vi "Add BPP Test Results Data new.vi"(8 "error in (no error)":errorcluster, 10 "Collimation Data":T1, 11 "Test in":refnum<k24>) -> (0 "error out":errorcluster, 3 "Test out":refnum<k24>)   [LabVIEW 2018]
uses:
  C:/Program Files (x86)/National Instruments/LabVIEW 2018/user.lib/nEQdb_DLL/NEQdbAPI.dll
  Program Files (x86)/National Instruments/LabVIEW 2018/user.lib/nEQdb_DLL/NEQdbAPI.dll
  State data/Records.ctl
  0415c7d9-6818-4349-a3d2-afeb8a82f6ab.vi
  0415c7d9-6818-4349-a3d2-afeb8a82f6ab.vi/6e08599f-9911-4127-abcd-496574c18721.vi
panel:
  in  "BPP items to save":T2(ring)
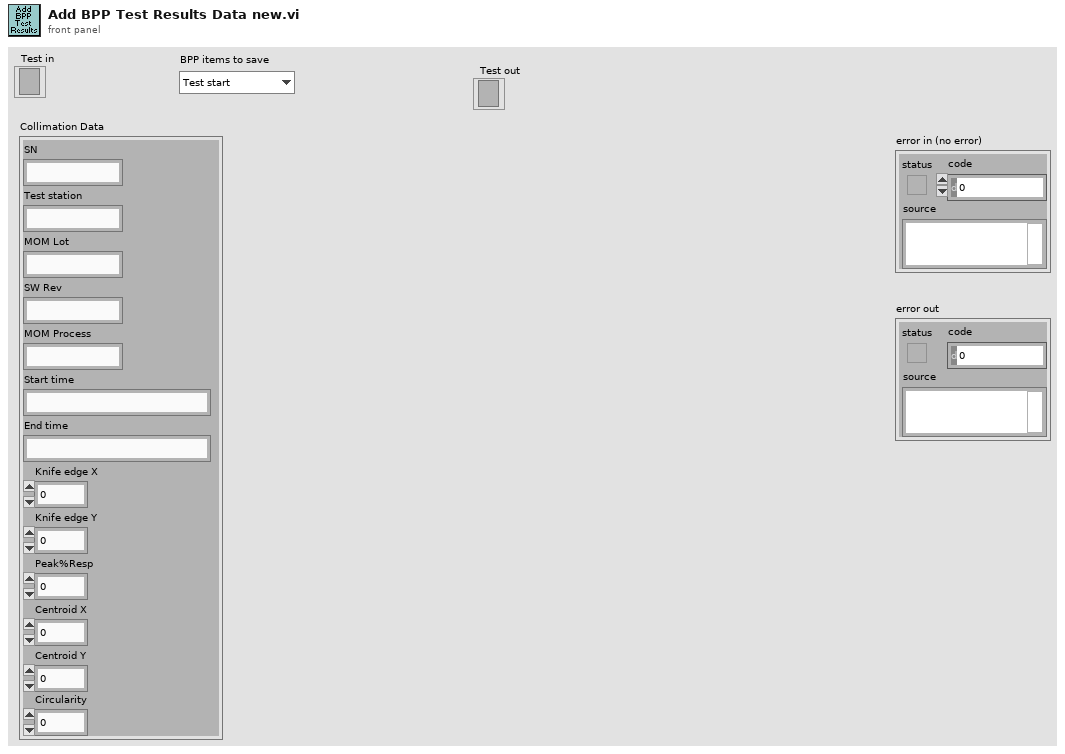
[diagram p1: front panel]
types:
  T1 = typedef "Records.ctl" = cluster{"SN":string, "Test station":string, "MOM Lot":string, "SW Rev":string, "MOM Process":string, "Start time":string, "End time":string, "Knife edge X":dbl, "Peak%Resp":dbl, "Centroid X":dbl, "Knife edge Y":dbl, "Centroid Y":dbl, "Circularity":dbl}
  T2 = enum16{"Test start", "Test finish", "FF Peak Response", "Ellipticity", "MeasuredCentroidX", "MeasuredCentroidY", "BeamViewKnifeEdge84PctX", "BeamViewKnifeEdge84PctY"}
  T3 = enum16{"Test start", "Test finish", "FF Peak Response", "Ellipticity", "MeasuredCentroidX", "MeasuredCentroidY", "BeamViewKnifeEdge84PctX", "BeamViewKnifeEdge84PctY"}[]
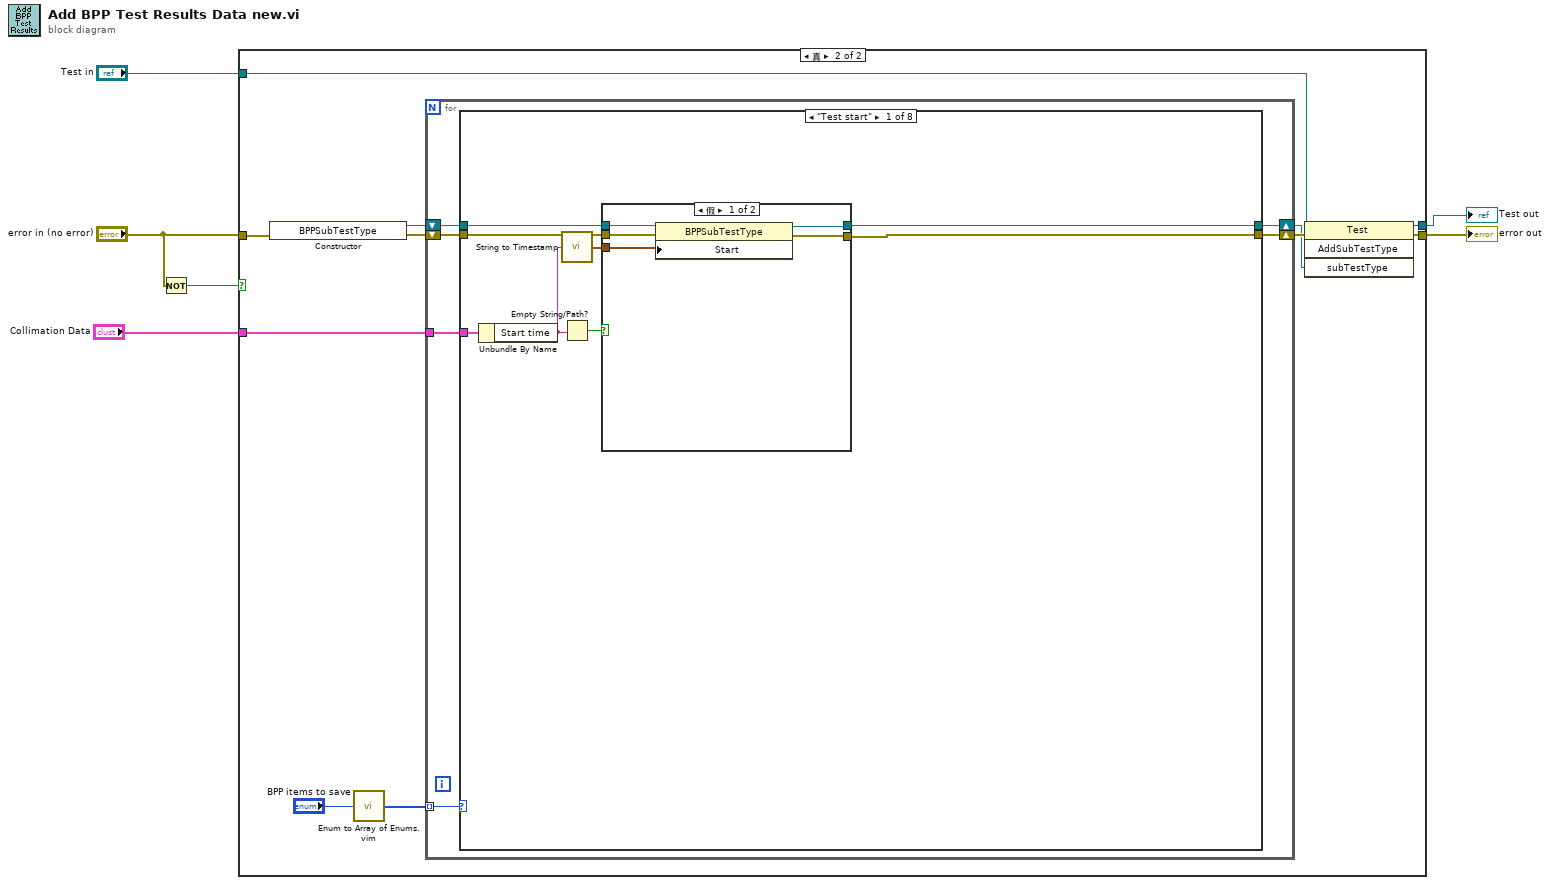
[diagram p0: block diagram]
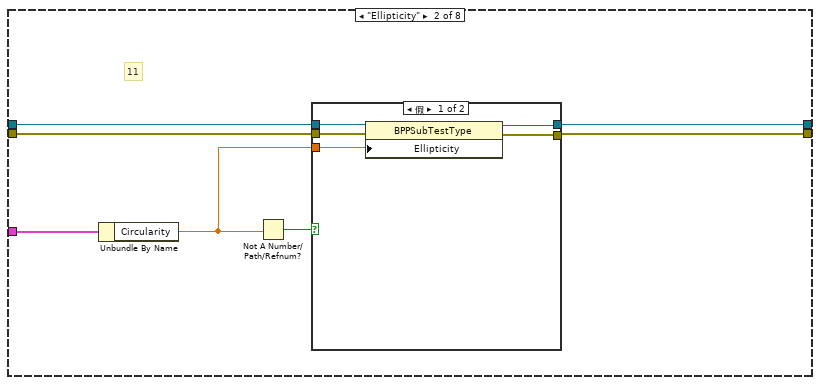
[diagram p4: hidden frame]
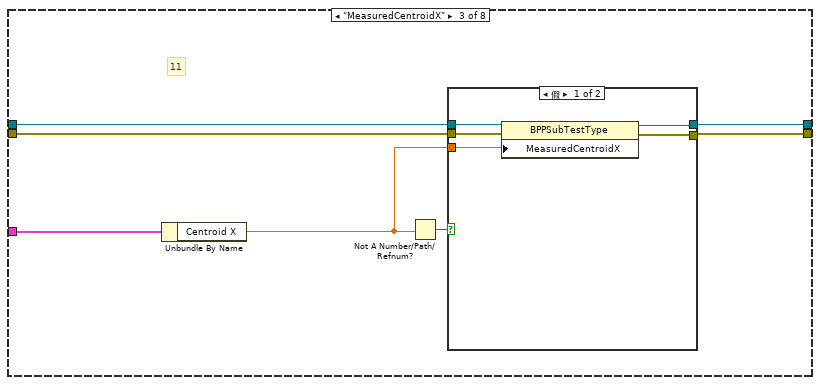
[diagram p6: hidden frame]
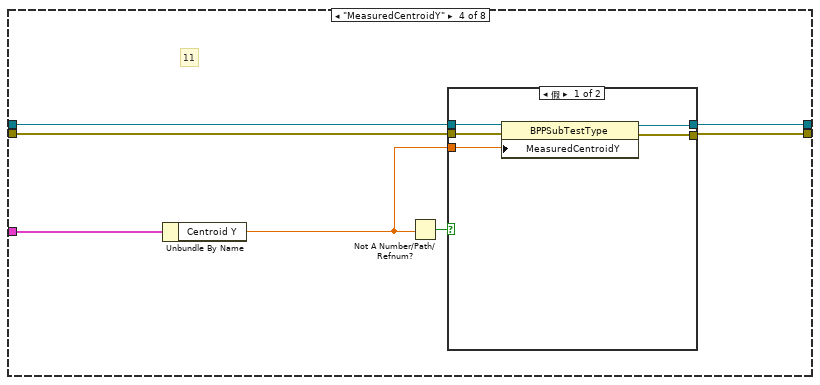
[diagram p8: hidden frame]
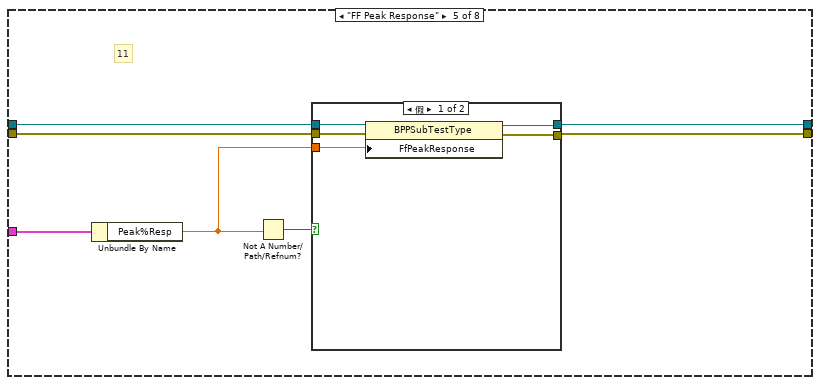
[diagram p10: hidden frame]
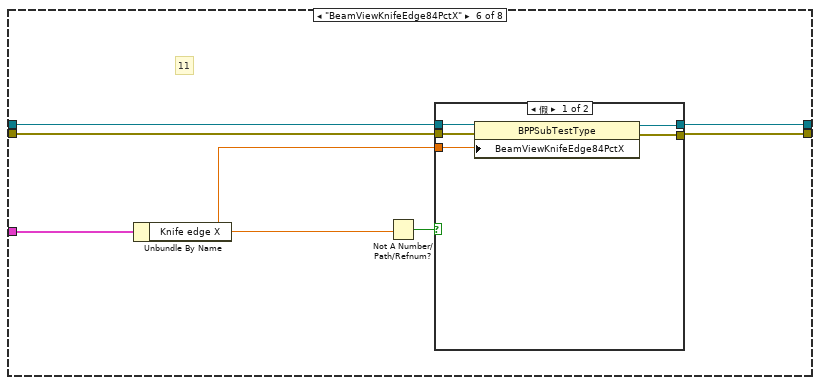
[diagram p12: hidden frame]
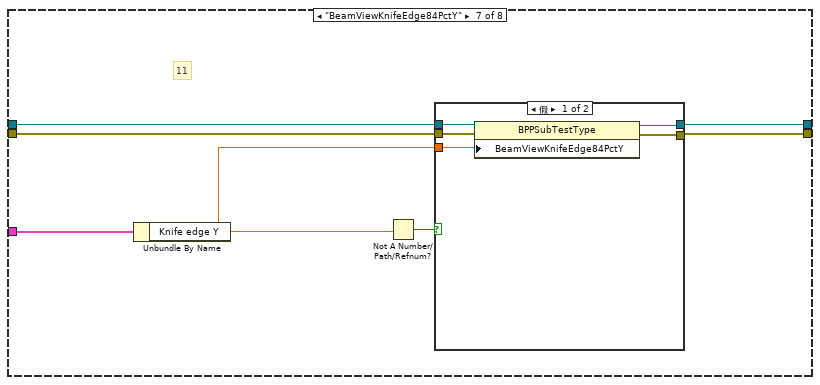
[diagram p14: hidden frame]
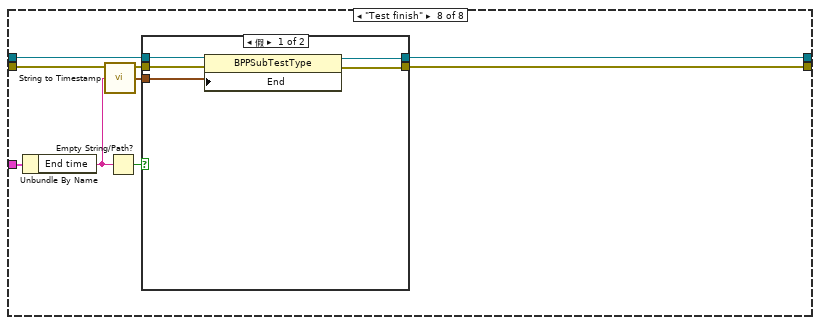
[diagram p16: hidden frame]
diagram:
  n1 = Not(x="error in (no error)") -> (.not. x?=w1:bool)
  n2 = case shown="真" w1 {
    tunnel: "Collimation Data" -> [_ w12]
    tunnel: "Test in" -> [w8 w16]
    tunnel: [w8 w14] -> w3
    tunnel: [w7 w13] -> w6
    tunnel: "error in (no error)" -> [w7 w19]
    frame False {
    }
    frame True {
      n3 = constructor class="BPPSubTestType"(error in=w19) -> (reference out=w18:refnum<k24>, error out=w17:errorcluster)  [unwired: 2 in, 1 out]
      n4 = call "Enum to Array of Enums.vim"("enum"="BPP items to save") -> ("array of enums"=w9:T3)
      n5 = for {
        shift-right: [w23] -> w15
        shift-left: w17 -> [w24]
        tunnel: w12 -> [w22]
        shift-right: [w21] -> w11
        shift-left: w18 -> [w25]
        tunnel: w9 -> [w20] mode=indexing
        n6 = case shown="\"Test start\"" w20 {
          tunnel: w25 -> [w31 w45 w59 w73 w87 w101 w115 w130]
          tunnel: w24 -> [w28 w42 w56 w70 w84 w98 w112 w128]
          tunnel: [w29 w43 w57 w71 w85 w99 w113 w127] -> w23
          tunnel: [w30 w44 w58 w72 w86 w100 w114 w129] -> w21
          tunnel: w22 -> [w33 w47 w61 w75 w89 w103 w117 w132]
          frame "Test start" {
            n7 = Unbundle By Name(w33) -> ("Start time"=w27:string)
            n8 = call <userlib>:"String to Timestamp.vi"("String for time conversion"=w27) -> ("Time Stamp"=w26:timestamp)
            n9 = Empty String/Path?(string/path=w27) -> (empty?=w32:bool)
            n10 = case shown="假" w32 {
              tunnel: w31 -> [w38 w40]
              tunnel: [w35 w40] -> w30
              tunnel: [w34 w39] -> w29
              tunnel: w28 -> [w37 w39]
              tunnel: w26 -> [w36 _]
              frame False {
                n11 = property on="属性节点" class="BPPSubTestType"(reference=w38, error in=w37, "Start"=w36) -> (reference out=w35:refnum<k24>, error out=w34:errorcluster)
              }
              frame True {
              }
            }
          }
          frame "Ellipticity" {
            # "11"
            n12 = Unbundle By Name(w47) -> ("Circularity"=w41:dbl)
            n13 = Not A Number/Path/Refnum?(number/path/refnum=w41) -> (NaN/Path/Refnum?=w46:bool)
            n14 = case shown="假" w46 {
              tunnel: w45 -> [w52 w54]
              tunnel: [w50 w54] -> w44
              tunnel: [w49 w53] -> w43
              tunnel: w42 -> [w51 w53]
              tunnel: w41 -> [w48 _]
              frame False {
                n15 = property on="属性节点" class="BPPSubTestType"(reference=w52, error in=w51, "Ellipticity"=w48) -> (reference out=w50:refnum<k24>, error out=w49:errorcluster)
              }
              frame True {
              }
            }
          }
          frame "MeasuredCentroidX" {
            # "11"
            n16 = Unbundle By Name(w61) -> ("Centroid X"=w55:dbl)
            n17 = Not A Number/Path/Refnum?(number/path/refnum=w55) -> (NaN/Path/Refnum?=w60:bool)
            n18 = case shown="假" w60 {
              tunnel: w59 -> [w66 w68]
              tunnel: [w64 w68] -> w58
              tunnel: [w63 w67] -> w57
              tunnel: w56 -> [w65 w67]
              tunnel: w55 -> [w62 _]
              frame False {
                n19 = property on="属性节点" class="BPPSubTestType"(reference=w66, error in=w65, "MeasuredCentroidX"=w62) -> (reference out=w64:refnum<k24>, error out=w63:errorcluster)
              }
              frame True {
              }
            }
          }
          frame "MeasuredCentroidY" {
            # "11"
            n20 = Unbundle By Name(w75) -> ("Centroid Y"=w69:dbl)
            n21 = Not A Number/Path/Refnum?(number/path/refnum=w69) -> (NaN/Path/Refnum?=w74:bool)
            n22 = case shown="假" w74 {
              tunnel: w73 -> [w80 w82]
              tunnel: [w78 w82] -> w72
              tunnel: [w77 w81] -> w71
              tunnel: w70 -> [w79 w81]
              tunnel: w69 -> [w76 _]
              frame False {
                n23 = property on="属性节点" class="BPPSubTestType"(reference=w80, error in=w79, "MeasuredCentroidY"=w76) -> (reference out=w78:refnum<k24>, error out=w77:errorcluster)
              }
              frame True {
              }
            }
          }
          frame "FF Peak Response" {
            # "11"
            n24 = Unbundle By Name(w89) -> ("Peak%Resp"=w83:dbl)
            n25 = Not A Number/Path/Refnum?(number/path/refnum=w83) -> (NaN/Path/Refnum?=w88:bool)
            n26 = case shown="假" w88 {
              tunnel: w87 -> [w94 w96]
              tunnel: [w92 w96] -> w86
              tunnel: [w91 w95] -> w85
              tunnel: w84 -> [w93 w95]
              tunnel: w83 -> [w90 _]
              frame False {
                n27 = property on="属性节点" class="BPPSubTestType"(reference=w94, error in=w93, "FfPeakResponse"=w90) -> (reference out=w92:refnum<k24>, error out=w91:errorcluster)
              }
              frame True {
              }
            }
          }
          frame "BeamViewKnifeEdge84PctX" {
            # "11"
            n28 = Unbundle By Name(w103) -> ("Knife edge X"=w97:dbl)
            n29 = Not A Number/Path/Refnum?(number/path/refnum=w97) -> (NaN/Path/Refnum?=w102:bool)
            n30 = case shown="假" w102 {
              tunnel: w101 -> [w108 w110]
              tunnel: [w106 w110] -> w100
              tunnel: [w105 w109] -> w99
              tunnel: w98 -> [w107 w109]
              tunnel: w97 -> [w104 _]
              frame False {
                n31 = property on="属性节点" class="BPPSubTestType"(reference=w108, error in=w107, "BeamViewKnifeEdge84PctX"=w104) -> (reference out=w106:refnum<k24>, error out=w105:errorcluster)
              }
              frame True {
              }
            }
          }
          frame "BeamViewKnifeEdge84PctY" {
            # "11"
            n32 = Unbundle By Name(w117) -> ("Knife edge Y"=w111:dbl)
            n33 = Not A Number/Path/Refnum?(number/path/refnum=w111) -> (NaN/Path/Refnum?=w116:bool)
            n34 = case shown="假" w116 {
              tunnel: w115 -> [w122 w124]
              tunnel: [w120 w124] -> w114
              tunnel: [w119 w123] -> w113
              tunnel: w112 -> [w121 w123]
              tunnel: w111 -> [w118 _]
              frame False {
                n35 = property on="属性节点" class="BPPSubTestType"(reference=w122, error in=w121, "BeamViewKnifeEdge84PctY"=w118) -> (reference out=w120:refnum<k24>, error out=w119:errorcluster)
              }
              frame True {
              }
            }
          }
          frame "Test finish" {
            n36 = Unbundle By Name(w132) -> ("End time"=w126:string)
            n37 = call <userlib>:"String to Timestamp.vi"("String for time conversion"=w126) -> ("Time Stamp"=w125:timestamp)
            n38 = Empty String/Path?(string/path=w126) -> (empty?=w131:bool)
            n39 = case shown="假" w131 {
              tunnel: [w135 w139] -> w129
              tunnel: w130 -> [w137 w139]
              tunnel: [w134 w138] -> w127
              tunnel: w128 -> [w136 w138]
              tunnel: w125 -> [w133 _]
              frame False {
                n40 = property on="属性节点" class="BPPSubTestType"(reference=w137, error in=w136, "End"=w133) -> (reference out=w135:refnum<k24>, error out=w134:errorcluster)
              }
              frame True {
              }
            }
          }
        }
      }
      n41 = invoke class="Test" method="AddSubTestType"(reference=w16, error in=w15, "subTestType"=w11) -> (reference out=w14:refnum<k24>, error out=w13:errorcluster)  [unwired: 1 in, 2 out]
    }
  }
  "error out" <- w6
  "Test out" <- w3
